vi "ControlTimersGLOBAL (1).vi"() -> ()   [LabVIEW 2017]
panel:
  in  "EndCoast":i64
  in  "EndPush":i64
  in  "CurrentTime":i64
  in  "StartPush":i64
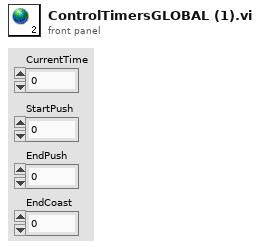
[diagram p1: front panel]
diagram:
